vi "Extract3ColumnsStorage.vi"(8 "Error In":errorcluster, 11 "Input Array":string[][](array[string])) -> (0 "Error Out":errorcluster, 1 "Filtered Array Out":string[][](array[string]), 2 "Property Out":string[](array[string]), 3 "Unit Out":string[](array[string]))   [LabVIEW 2014]
uses:
  Controls/ColumnHeaders1.ctl
  <userlib>/_RADE/MTA-lib/array/array.llb/Search 1D Array (String)__ogtk.vi
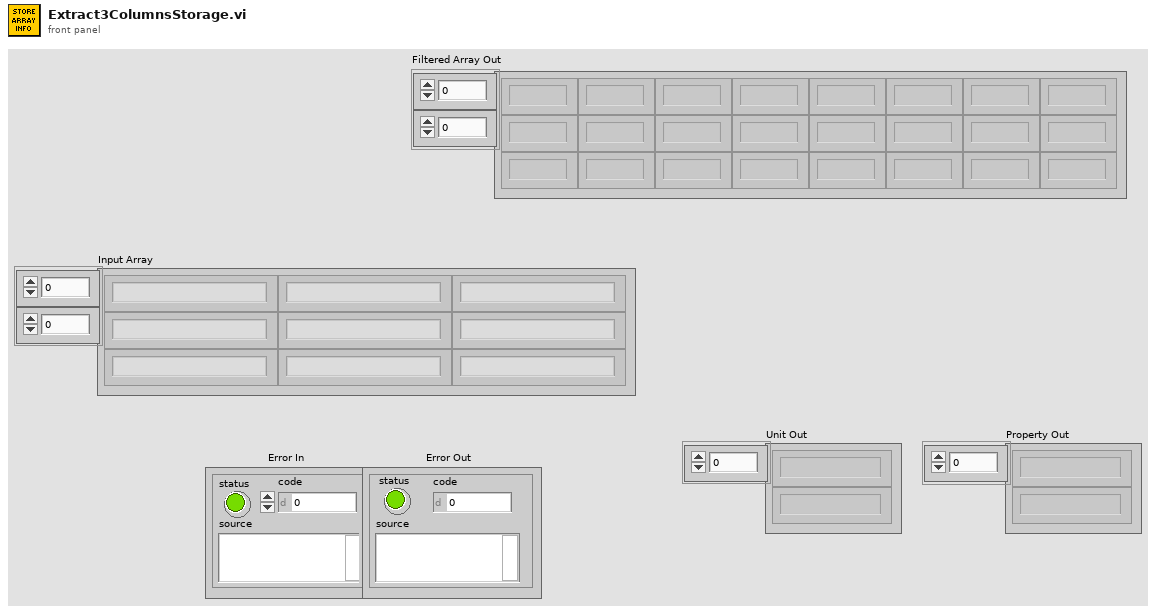
[diagram p1: front panel]
types:
  T1 = typedef "ColumnHeaders1.ctl" = enum16{"Store", "Display", "Method", "Property", "Unit", "URL", "IP Address", "Data Block", "Address", "Data Type"}
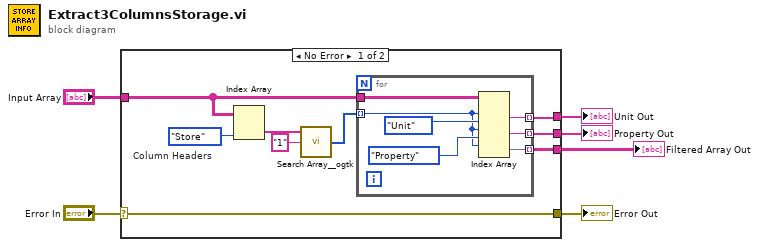
[diagram p0: block diagram]
diagram:
  n1 = case shown="No Error" "Error In" {
    selector: "Error In" -> [w15 w23]
    tunnel: [w15 w23] -> w6
    tunnel: "Input Array" -> [w8 _]
    tunnel: [w11 _] -> w3
    tunnel: [w10 _] -> w2
    tunnel: [w7 _] -> w1
    frame No Error {
      w14 = ColumnHeaders1."Store"  # Column Headers
      n2 = Index Array(array=w8, index (col)=w14) -> (element=w13:string[])  [unwired: 1 in]
      n3 = call-poly <userlib>:"Search Array__ogtk.vi"("Array"=w13, "Element Data"="1") -> ("Indices of Elements"=w12:i32[])  [unwired: 7 in]
      n4 = for {
        tunnel: w8 -> [w22]
        tunnel: w12 -> [w17] mode=indexing
        tunnel: [w19] -> w11 mode=indexing
        tunnel: [w18] -> w10 mode=indexing
        tunnel: [w16] -> w7 mode=indexing
        n5 = Index Array(array=w22, index (row) #1=w17, index (col) #1=ColumnHeaders1."Unit" ("Property 2"), index (row) #2=w17, index (col) #2=ColumnHeaders1."Property" ("Property 2"), index (row) #3=w17) -> (element #1=w19:string, element #2=w18:string, element #3=w16:string[])  [unwired: 1 in]
      }
    }
    frame Error {
    }
  }
  "Error Out" <- w6
  "Property Out" <- w2
  "Unit Out" <- w3
  "Filtered Array Out" <- w1
